vi "Deadband Checker.vi"(10 "Limit":dbl, 11 "Value":dbl) -> (3 "Outside Deadband?":bool)   [LabVIEW 2023]
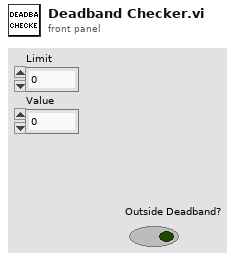
[diagram p1: front panel]
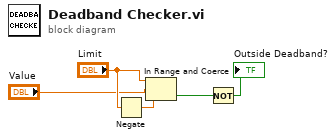
[diagram p0: block diagram]
diagram:
  n1 = Negate(x="Limit") -> (-x=w3:dbl)
  n2 = In Range and Coerce(upper limit="Limit", x="Value", lower limit=w3) -> (In Range?=w4:bool)  [unwired: 1 out]
  n3 = Not(x=w4) -> (.not. x?=→"Outside Deadband?":bool)
